vi "Simulate hardware.vi"() -> ()   [LabVIEW 2020]
uses:
  <vilib>/DAQmx/read.llb/DAQmx Read (Analog Wfm 1Chan NSamp).vi
  <vilib>/DAQmx/create/channels.llb/DAQmx Create Channel (AI-Voltage-Basic).vi
  <vilib>/DAQmx/configure/timing.llb/DAQmx Timing (Sample Clock).vi
  <vilib>/DAQmx/miscellaneous.llb/DAQmx Fill In Error Info.vi
panel:
  out "Waveform Chart 2":waveform(dbl)(graph)
  out "error out 2":errorcluster
  in  "error in 2":errorcluster
  in  "stop":bool
  in  "error in":errorcluster
  out "error out":errorcluster
  out "Waveform Chart":waveform(dbl)(graph)
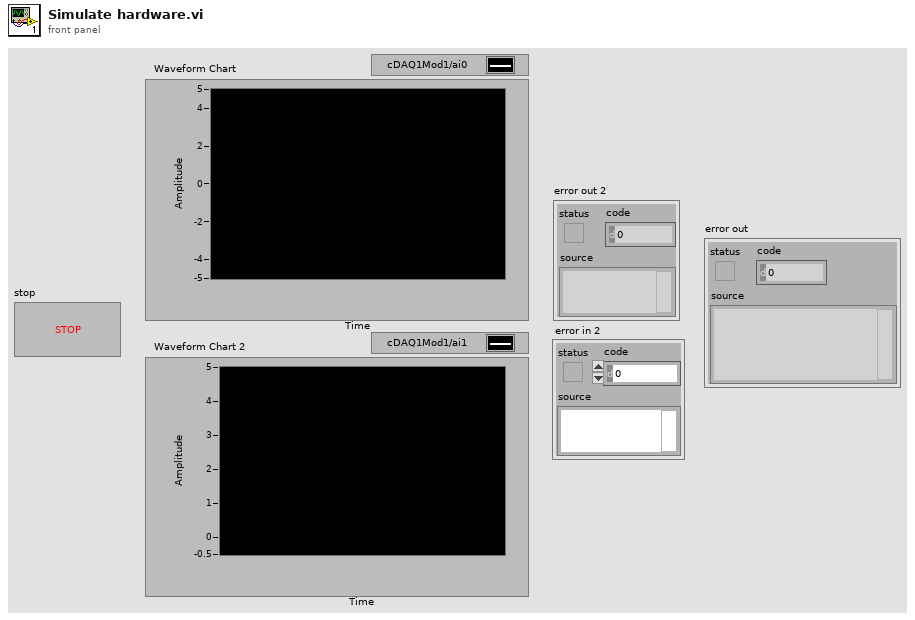
[diagram p1: front panel]
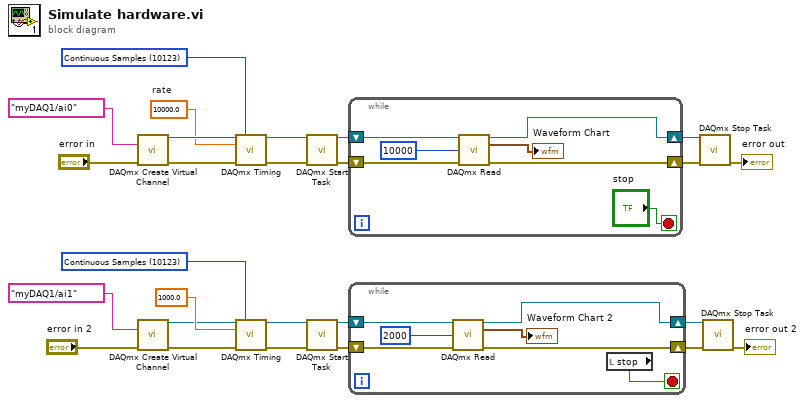
[diagram p0: block diagram]
diagram:
  w13 = 10123 items=["Finite Samples"=10178, "Continuous Samples"=10123, "Hardware Timed Single Point"=12522] ("sample mode")
  w14 = 10123 items=["Finite Samples"=10178, "Continuous Samples"=10123, "Hardware Timed Single Point"=12522] ("sample mode")
  w15 = 10000.0  # rate
  n1 = call-poly <vilib>:"DAQmx Create Virtual Channel.vi"("physical channels"=tag "myDAQ1/ai0", "error in"="error in") -> ("task out"=w22:refnum<k21>, "error out"=w21:errorcluster)  [unwired: 12 in]
  n2 = call-poly <vilib>:"DAQmx Create Virtual Channel.vi"("physical channels"=tag "myDAQ1/ai1", "error in"="error in 2") -> ("task out"=w5:refnum<k21>, "error out"=w6:errorcluster)  [unwired: 12 in]
  n3 = call-poly <vilib>:"DAQmx Timing.vi"("task/channels in"=w22, "sample mode"=w14, "rate"=w15, "error in"=w21) -> ("task out"=w24:refnum<k21>, "error out"=w23:errorcluster)  [unwired: 10 in]
  n4 = call-poly <vilib>:"DAQmx Timing.vi"("task/channels in"=w5, "sample mode"=w13, "rate"=1000.0, "error in"=w6) -> ("task out"=w3:refnum<k21>, "error out"=w4:errorcluster)  [unwired: 10 in]
  n5 = call <vilib>:"DAQmx Start Task.vi"("task/channels in"=w24, "error in"=w23) -> ("task out"=w26:refnum<k21>, "error out"=w25:errorcluster)  [unwired: 12 in]
  n6 = call <vilib>:"DAQmx Start Task.vi"("task/channels in"=w3, "error in"=w4) -> ("task out"=w1:refnum<k21>, "error out"=w2:errorcluster)  [unwired: 12 in]
  n7 = while {
    shift-right: [w31] -> w19
    shift-left: w26 -> [w33]
    shift-right: [w30] -> w18
    shift-left: w25 -> [w32]
    stop <- "stop" stop-if-true
    n8 = call-poly <vilib>:"DAQmx Read.vi"("task/channels in"=w33, "number of samples per channel"=10000, "error in"=w32) -> ("task out"=w31:refnum<k21>, "data"=→"Waveform Chart":waveform(dbl), "error out"=w30:errorcluster)  [unwired: 10 in]
  }
  n9 = while {
    shift-right: [w38] -> w8
    shift-left: w1 -> [w40]
    shift-right: [w37] -> w9
    shift-left: w2 -> [w39]
    stop <- w35 stop-if-true
    n10 = call-poly <vilib>:"DAQmx Read.vi"("task/channels in"=w40, "number of samples per channel"=2000, "error in"=w39) -> ("task out"=w38:refnum<k21>, "data"=→"Waveform Chart 2":waveform(dbl), "error out"=w37:errorcluster)  [unwired: 10 in]
    n11 = local read "stop"() -> (w35:bool)
  }
  n12 = call <vilib>:"DAQmx Stop Task.vi"("task/channels in"=w19, "error in"=w18) -> ("error out"=→"error out":errorcluster)  [unwired: 12 in, 1 out]
  n13 = call <vilib>:"DAQmx Stop Task.vi"("task/channels in"=w8, "error in"=w9) -> ("error out"=→"error out 2":errorcluster)  [unwired: 12 in, 1 out]
